vi "BRig_Host__Loop_Consumer_AnalogInput__parse.vi"(11 "input_strCmd":string) -> (0 "output_ai1":i32, 1 "output_ai0":i32, 3 "output_haveAnalogInput":bool)   [LabVIEW 2014]
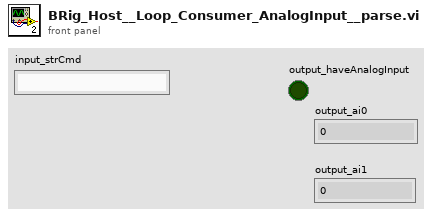
[diagram p1: front panel]
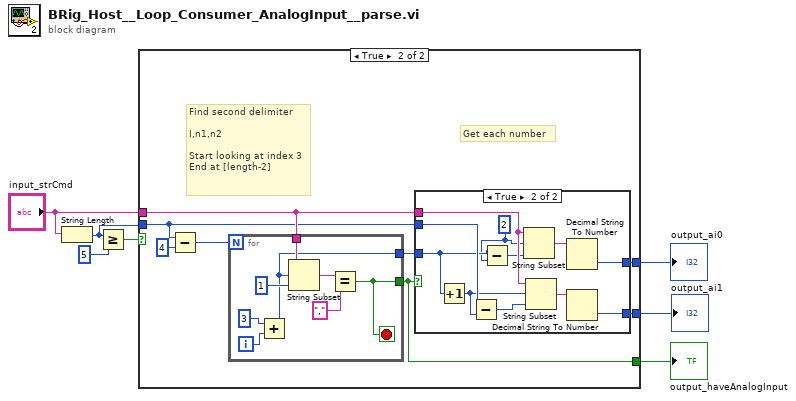
[diagram p0: block diagram]
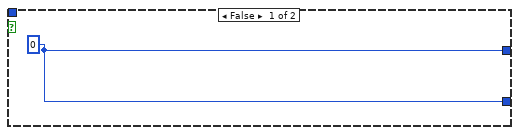
[diagram p2: hidden frame]
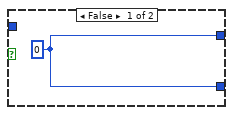
[diagram p3: hidden frame]
diagram:
  n1 = String Length(string="input_strCmd") -> (length=w6:i32)
  n2 = Greater Or Equal?(x=w6, y=5) -> (x >= y?=w4:bool)
  n3 = case shown="True" w4 {
    tunnel: w6 -> [_ w12]
    tunnel: "input_strCmd" -> [_ w13]
    tunnel: [w8 w11] -> w3
    tunnel: [w8 w10] -> w2
    tunnel: [_ w9] -> w1
    frame False {
      w8 = 0
    }
    frame True {
      # "Get each number"
      # "Find second delimiter\n\nI,n1,n2\n\nStart looking at index 3\nEnd at [length-2]"
      n4 = Subtract(x=w12, y=4) -> (x-y=w15:i32)
      n5 = for {
        N: w15 -> [_]
        tunnel: w13 -> [w34]
        tunnel: [w30] -> w9
        tunnel: [w29] -> w14
        i -> [w36]
        stop <- w30 stop-if-true
        n6 = Add(x=3 ("y"), y=w36) -> (x+y=w29:i32)
        n7 = String Subset(string=w34, offset (0)=w29, length (rest)=1 ("length (rest)")) -> (substring=w32:string)
        n8 = Equal?(x=w32, y=",") -> (x = y?=w30:bool)
      }
      n9 = case shown="True" w9 {
        tunnel: w14 -> [_ w19]
        tunnel: w13 -> [_ w28]
        tunnel: w12 -> [_ w26]
        tunnel: [w17 w21] -> w11
        tunnel: [w17 w20] -> w10
        frame False {
          w17 = 0
        }
        frame True {
          w18 = 2 ("y")
          n10 = Increment(x=w19) -> (x+1=w24:i32)
          n11 = Subtract(x=w26, y=w24) -> (x-y=w25:i32)
          n12 = Subtract(x=w19, y=w18) -> (x-y=w27:i32)
          n13 = String Subset(string=w28, offset (0)=w18, length (rest)=w27) -> (substring=w23:string)
          n14 = String Subset(string=w28, offset (0)=w24, length (rest)=w25) -> (substring=w22:string)
          n15 = Decimal String To Number(string=w23) -> (number=w21:i32)  [unwired: 2 in, 1 out]
          n16 = Decimal String To Number(string=w22) -> (number=w20:i32)  [unwired: 2 in, 1 out]
        }
      }
    }
  }
  "output_haveAnalogInput" <- w1
  "output_ai0" <- w3
  "output_ai1" <- w2
